vi "readphoto.vi"(6 "name or relative path":path) -> (5 "dataOut":string)   [LabVIEW 2021]
panel:
  out "fileName":string
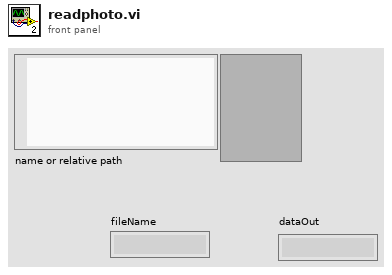
[diagram p1: front panel]
types:
  T1 = enum16{"open", "replace", "create", "open or create", "replace or create", "replace or create with confirmation"}
  T2 = enum16{"big-endian, network order", "native, host order", "little-endian"}
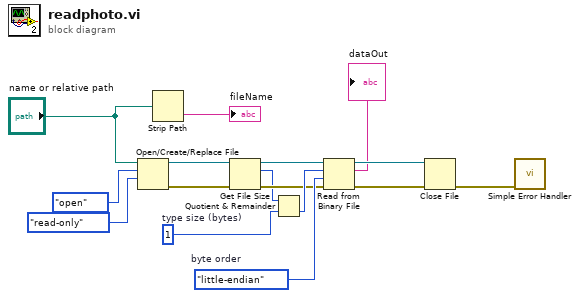
[diagram p0: block diagram]
diagram:
  w12 = T2."little-endian"  # byte order
  w10 = i64 1  # type size (bytes)
  n1 = Open/Create/Replace File(file path (use dialog)="name or relative path", operation (0:open)=T1."open", access (0:read/write)=enum16{"read/write", "read-only", "write-only"}."read-only") -> (refnum out=w15:refnum<file>, error out=w14:errorcluster)  [unwired: 3 in, 1 out]
  n2 = Strip Path(path="name or relative path") -> (name=→"fileName":string)  [unwired: 1 out]
  n3 = Get File Size(file=w15, error in=w14) -> (refnum out=w4:refnum<file>, size (in bytes)=w7:i64, 0:w8:errorcluster)
  n4 = Quotient & Remainder(x=w7, y=w10) -> (floor(x/y)=w11:i64)  [unwired: 1 out]
  n5 = Read from Binary File(8:w8, 9:w12, 10:w11, 11:w4) -> (0:w6:errorcluster, 2:→"dataOut":string, 3:w5:refnum<file>)  [unwired: 2 in, 1 out]
  n6 = Close File(refnum=w5, error in=w6) -> (error out=w16:errorcluster)  [unwired: 1 out]
  n7 = call <vilib>:"Simple Error Handler.vi"("error in (no error)"=w16) -> ()  [unwired: 4 in, 5 out]
